vi "Get predef instructions.vi"(8 "error in (no error)":errorcluster, 11 "Motor in":refnum<class "Motor.lvclass">) -> (0 "error out":errorcluster, 2 "instructions":string[](array[string]), 3 "Motor out":refnum<class "Motor.lvclass">)   [LabVIEW 2018, in "Motor.lvclass"]
uses:
  Motor.lvclass
  Motor.lvclass/Motor.ctl
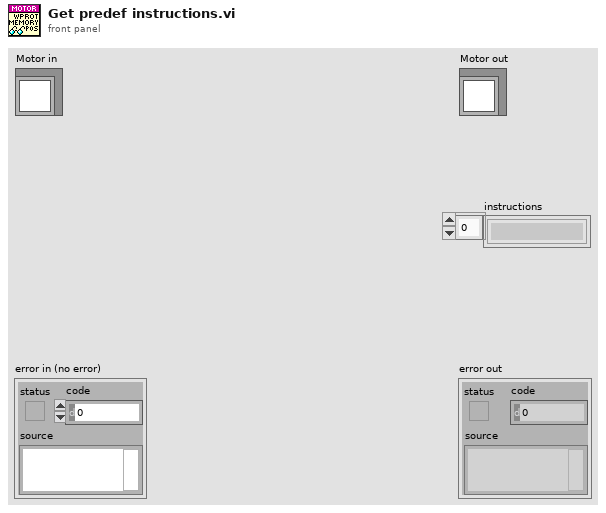
[diagram p1: front panel]
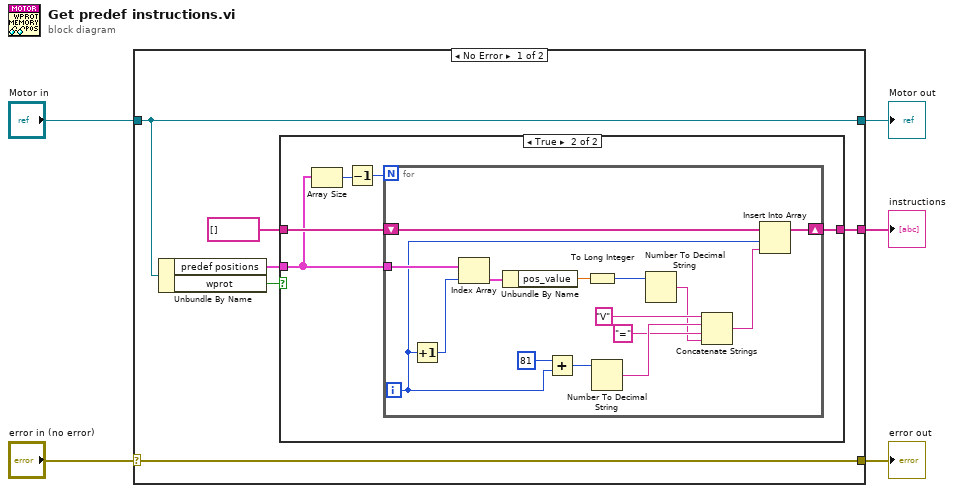
[diagram p0: block diagram]
diagram:
  n1 = case shown="No Error" "error in (no error)" {
    selector: "error in (no error)" -> [w11 w33]
    tunnel: [w11 w33] -> w4
    tunnel: [w10 w34] -> w2
    tunnel: "Motor in" -> [w10 w34]
    tunnel: [w7 _] -> w1
    frame No Error {
      n2 = Unbundle By Name(w10) -> ("predef positions"=w8:cluster{"pos_name":string, "pos_value":dbl}[], "wprot"=w9:bool)
      n3 = case shown="True" w9 {
        tunnel: w8 -> [_ w15]
        tunnel: [w12 w17] -> w7
        tunnel: string[] [] ("appended array") -> [w12 w16]
        frame False {
        }
        frame True {
          n4 = Array Size(array=w15) -> (size(s)=w14:i32)
          n5 = Decrement(x=w14) -> (x-1=w13:i32)
          n6 = for {
            N: w13 -> [_]
            tunnel: w15 -> [w21]
            shift-right: [w24] -> w17
            shift-left: w16 -> [w25]
            i -> [w18]
            n7 = Increment(x=w18) -> (x+1=w20:i32)
            n8 = Index Array(array=w21, index=w20) -> (element=w19:cluster{"pos_name":string, "pos_value":dbl})
            n9 = Unbundle By Name(w19) -> ("pos_value"=w31:dbl)
            n10 = Add(x=81, y=w18) -> (x+y=w29:i32)
            n11 = To Long Integer(number=w31) -> (32bit integer=w32:i32)
            n12 = Number To Decimal String(number=w29) -> (decimal integer string=w27:string)  [unwired: 1 in]
            n13 = Number To Decimal String(number=w32) -> (decimal integer string=w22:string)  [unwired: 1 in]
            n14 = Concatenate Strings("V" ("string"), w27, "=" ("string"), w22) -> (w23:string)
            n15 = Insert Into Array(array=w25, index=w18, new element=w23) -> (w24:string[])
          }
        }
      }
    }
    frame Error {
    }
  }
  "error out" <- w4
  "Motor out" <- w2
  "instructions" <- w1
